vi "Untitled 5.vi"() -> ()   [LabVIEW 2019]
uses:
  <vilib>/Platform/TimedLoop/XDataNode/wakeup.ctl
  <vilib>/Platform/TimedLoop/XDataNode/XDNodeRunTimeDep.lvlib
  <vilib>/Platform/TimedLoop/XDataNode/nitl_modes.ctl
  <vilib>/Platform/TimedLoop/XDataNode/timing_clust.ctl
  <vilib>/Platform/TimedLoop/XDataNode/XDataNode.xnode
  <vilib>/rvi/DataTransferAndStorage/Container/XNode/niFpgaContainer.xnode
  Templates/FPGA Wizard Templates.lvlib
  <vilib>/rvi/interface/RandomDataEmulation/nirviRandomDataFpgaReadWriteTemplate.vi
  <vilib>/NI/Engine Simulation Toolkit (EST)/APU/Shared Settings.ctl
  <vilib>/NI/Engine Simulation Toolkit (EST)/Version Token.ctl
  <vilib>/NI/Engine Simulation Toolkit (EST)/APU/Settings.ctl
  <vilib>/NI/Engine Simulation Toolkit (EST)/APU/Input.ctl
  <vilib>/NI/Engine Simulation Toolkit (EST)/APU/Output.ctl
  <vilib>/NI/Engine Simulation Toolkit (EST)/Analog Replay/Load Input.ctl
  <vilib>/NI/Engine Simulation Toolkit (EST)/Digital Pattern Generation/Load Input.ctl
  <vilib>/NI/Engine Simulation Toolkit (EST)/Directional Speed/Load Input.ctl
panel:
  out "Numeric":fxp<+/-,32,8> format="%#_27g"
  out "Mod1.Monitor":fxp<+/-,24,5>[](array[numeric])
  in  "Crank":T1
  in  "Exhaust CAM":T2
  in  "Intake CAM":T2
  in  "VR Sensor":T3={"Data"=[0, 0, 0, 0, 0, 0, 0, 0, 0, 0, 0, 0, 0, 0, 0, 0], "LoadOffset"=0, "Done"=FALSE}
  in  "Analog Input Loop Timer (uSec)":u32
  out "output.apu 1":T4 caption="output"
  in  "input.apu 1":T5={"desired speed"=0.0, "reset"=TRUE} caption="input"
  in  "settings.apu 1":T6 caption="settings"
  in  "est.version":T7
  in  "shared settings.apu 1":T8 {"start" format="%#.15g"}
  in  "go.apu 1":bool
  in  "Digital Loop Timer (uSec)":u32
  in  "Analog Output Loop Timer (uSec)":u32
  in  "DMA.Enable":bool
  in  "DMA.MinimumSamples":u32 caption="DMA Loop Timer (uSec)"
  out "DMA.Timeout":bool
  in  "DMA.Timeout.Reset":bool
  in  "DMA Loop Timer (uSec)":u32
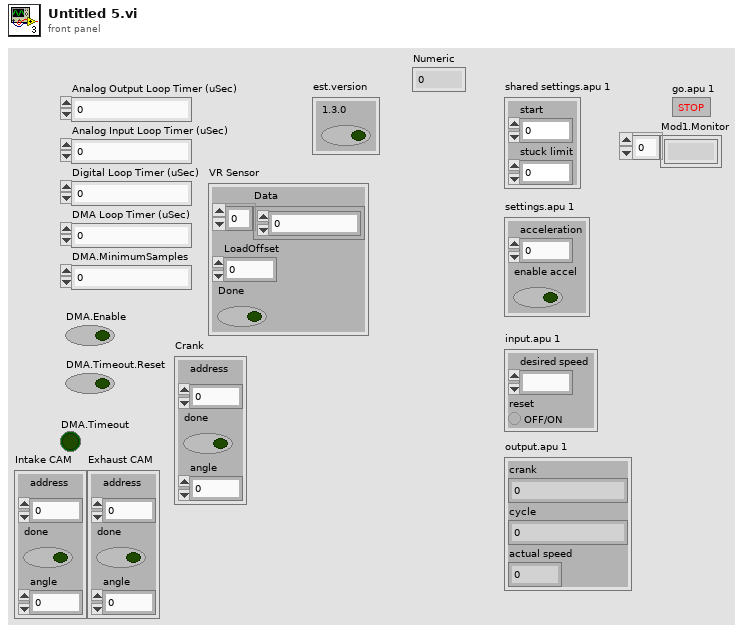
[diagram p1: front panel]
types:
  T1 = typedef "Engine Simulation Toolkit.lvlib/Directional Speed.lvlib/Load Input.ctl" = cluster{"address":fxp<+,10,10>, "done":bool, "angle":u16}
  T2 = typedef "Engine Simulation Toolkit.lvlib/Digital Pattern Generation.lvlib/Load Input.ctl" = cluster{"address":fxp<+,11,11>, "done":bool, "angle":u16}
  T3 = typedef "Engine Simulation Toolkit.lvlib/Analog Replay.lvlib/Load Input.ctl" = cluster{"Data":i16[], "LoadOffset":u16, "Done":bool}
  T4 = typedef "Engine Simulation Toolkit.lvlib/APU.lvlib/Output.ctl" = cluster{"crank":u16, "cycle":u16, "actual speed":fxp<+/-,23,2>}
  T5 = typedef "Engine Simulation Toolkit.lvlib/APU.lvlib/Input.ctl" = cluster{"desired speed":fxp<+/-,23,2>, "reset":bool}
  T6 = typedef "Engine Simulation Toolkit.lvlib/APU.lvlib/Settings.ctl" = cluster{"acceleration":fxp<+,18,-20>, "enable accel":bool}
  T7 = typedef "Engine Simulation Toolkit.lvlib/Version Token.ctl" = cluster{"1.3.0":bool}
  T8 = typedef "Engine Simulation Toolkit.lvlib/APU.lvlib/Shared Settings.ctl" = cluster{"start":fxp<+,17,17>, "stuck limit":fxp<+,18,18>}
  T9 = typedef "XDNodeRunTimeDep.lvlib/timing_clust.ctl" = cluster{"Expected End [f-1]":u64, "Actual End [f-1]":u64, "Finished Late? [f-1]":bool, "Expected End [i-1]":u64, "Actual End [i-1]":u64, "Finished Late? [i-1]":bool, "Expected Start [i]":u64, "Actual Start [i]":u64, "Expected Start [f]":u64, "Actual Start [f]":u64, "Source Name":string, "Structure Name":string, "Period":i64, "Deadline":i64, "Offset":i64, "Start":i64, "Priority":i32, "Timeout":i32, "Mode":T10, "Wakeup Reason":T11, "Error":errorcluster, "Source Type":string, "Secondary Source Type":string, "Global End Time":u64, "Global Start Time":u64, "Frame Duration":u64, "Iteration Duration":u64, "Assigned CPU":i32, "I/O Scan Engine Mode":u32}
  T10 = typedef "XDNodeRunTimeDep.lvlib/nitl_modes.ctl" = enum32{"No Change", "Process missed periods, maintain original phase", "Discard missed periods, maintain original phase", "Process missed periods, ignore original phase", "Discard missed periods, ignore original phase"}
  T11 = typedef "XDNodeRunTimeDep.lvlib/wakeup.ctl" = enum32{"Normal", "Aborted", "Asynchronous wakeup", "Timing source error", "Timed loop error", "Timeout"}
  T12 = cluster{"AI 0":refnum<k21>, "AI 1":refnum<k21>, "AI 2":refnum<k21>, "AI 3":refnum<k21>, "AI 4":refnum<k21>, "AI 5":refnum<k21>, "AI 6":refnum<k21>, "AI 7":refnum<k21>, "AI 8":refnum<k21>, "AI 9":refnum<k21>, "AI 10":refnum<k21>, "AI 11":refnum<k21>, "AI 12":refnum<k21>, "AI 13":refnum<k21>, "AI 14":refnum<k21>, "AI 15":refnum<k21>}
  T13 = typedef "Engine Simulation Toolkit.lvlib/APU.lvlib/Register Bus.ctl" = cluster{"Speed":refnum<k21>, "Crank Angle":refnum<k21>, "Cycle Angle":refnum<k21>, "Crank Count":refnum<k21>, "Cycle Count":refnum<k21>, "1.25 MHz Counter":refnum<k21>, "Crank Rollover":refnum<k21>, "Cycle Rollover":refnum<k21>, "shared settings":T8}
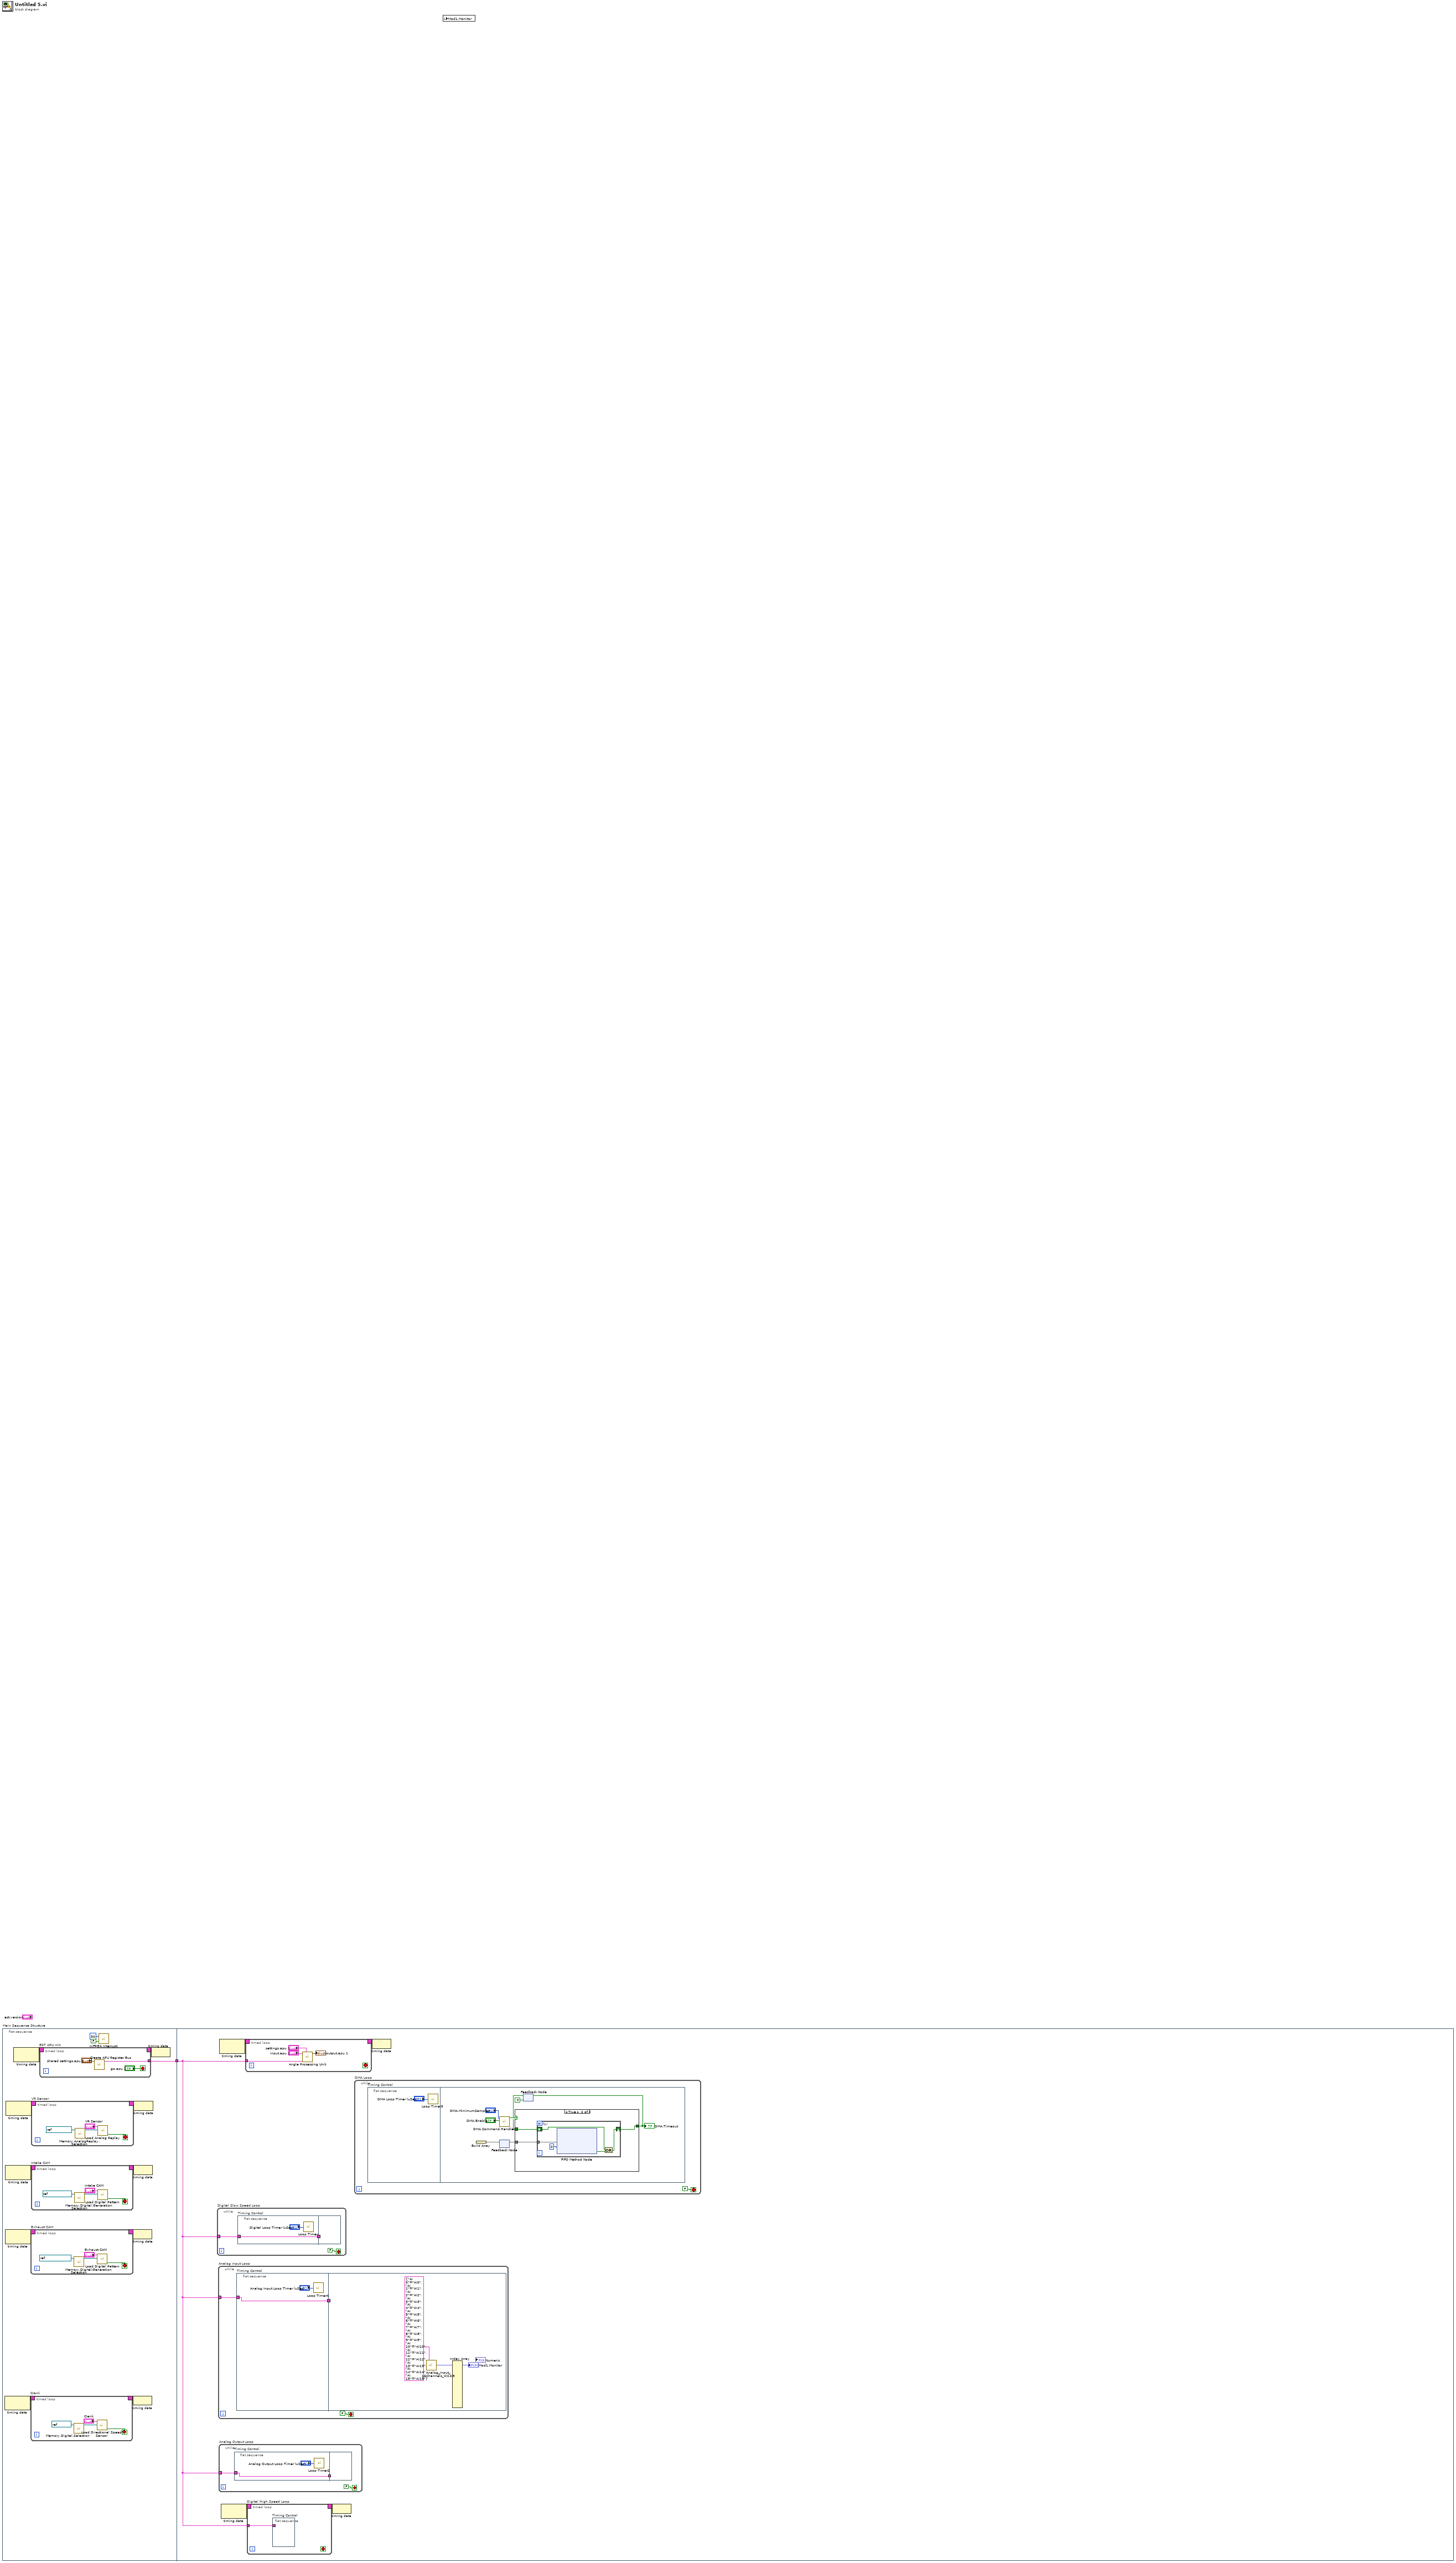
[diagram p0: block diagram]
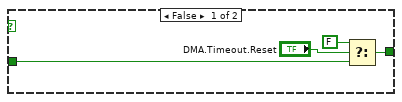
[diagram p2: hidden frame]
diagram:
  n1 = flat-sequence "Main Sequence Structure" {
    tunnel: [w10] -> w1
    tunnel: w1 -> [w54]
    frame #0 {
      n2 = node-c288() -> (w3:T9)  [unwired: 1 in]
      n3 = node-c288() -> (w5:T9)  [unwired: 1 in]
      n4 = node-c288() -> (w7:T9)  [unwired: 1 in]
      n5 = node-c288() -> (w9:T9)  [unwired: 1 in]
      n6 = node-c288() -> (w12:T9)  [unwired: 1 in]
      n7 = timed-loop "Crank" {
        timing: w3 -> [_]
        timing-out: [_] -> w2
        stop <- w17 stop-if-true
        n8 = call "Memory.Digital.Selection.vi"("memory"=refnum<k21> "Crank") -> ("memory"=w15:refnum<k21>)  [unwired: 10 in]
        n9 = call <vilib>:"Load Directional Speed Sensor.vi"("Memory In"=w15, "load input.<user name>"="Crank") -> ("done"=w17:bool)  [unwired: 8 in, 1 out]
      }
      n10 = timed-loop "Exhaust CAM" {
        timing: w5 -> [_]
        timing-out: [_] -> w4
        stop <- w25 stop-if-true
        n11 = call "Memory.Digital.Selection.vi"("memory"=refnum<k21> "Exhaust CAM") -> ("memory"=w23:refnum<k21>)  [unwired: 10 in]
        n12 = call <vilib>:"Load Digital Pattern Generation.vi"("memory"=w23, "load input.<user name>"="Exhaust CAM") -> ("done"=w25:bool)  [unwired: 8 in, 1 out]
      }
      n13 = timed-loop "Intake CAM" {
        timing: w7 -> [_]
        timing-out: [_] -> w6
        stop <- w33 stop-if-true
        n14 = call "Memory.Digital.Selection.vi"("memory"=refnum<k21> "Intake CAM") -> ("memory"=w31:refnum<k21>)  [unwired: 10 in]
        n15 = call <vilib>:"Load Digital Pattern Generation.vi"("memory"=w31, "load input.<user name>"="Intake CAM") -> ("done"=w33:bool)  [unwired: 8 in, 1 out]
      }
      n16 = timed-loop "VR Sensor" {
        timing: w9 -> [_]
        timing-out: [_] -> w8
        stop <- w41 stop-if-true
        n17 = call "Memory.AnalogReplay.Selection.vi"("memory"=refnum<k21> "VR Sensor") -> ("memory"=w39:refnum<k21>)  [unwired: 10 in]
        n18 = call <vilib>:"Load Analog Replay.vi"("memory"=w39, "load input.<user name>"="VR Sensor") -> ("done"=w41:bool)  [unwired: 9 in]
      }
      n19 = timed-loop "EST APU Init" {
        timing: w12 -> [_]
        timing-out: [_] -> w11
        tunnel: [w47] -> w10
        stop <- "go.apu 1" stop-if-true
        n20 = call <vilib>:"Create APU Register Bus.vi"("shared settings.<user name>"="shared settings.apu 1") -> ("register bus"=w47:T13)  [unwired: 10 in]
      }
      n21 = call <vilib>:"niFPGA Interrupt.vi"("Wait Until Cleared (F)"=FALSE, "IRQ Number (0)"=u8 30) -> ()  [unwired: 1 in]
      n22 = node-c288(w2) -> ()
      n23 = node-c288(w4) -> ()
      n24 = node-c288(w6) -> ()
      n25 = node-c288(w8) -> ()
      n26 = node-c288(w11) -> ()
    }
    frame #1 {
      # "FPGA Addon Code"
      n27 = while "Digital Slow Speed Loop" {
        tunnel: w54 -> [w107]
        stop <- FALSE stop-if-true
        n28 = flat-sequence "Timing Control" {
          tunnel: w107 -> [w109]
          tunnel: [w109] -> w106
          tunnel: w106 -> [_]
          frame #0 {
            n29 = call "Loop Timer"("Count(uSec)"="Digital Loop Timer (uSec)") -> ()  [unwired: 1 out]
          }
          frame #1 {
          }
        }
      }
      n30 = while "Analog Input Loop" {
        tunnel: w54 -> [w100]
        stop <- FALSE stop-if-true
        n31 = flat-sequence "Timing Control" {
          tunnel: w100 -> [w102]
          tunnel: [w102] -> w99
          tunnel: w99 -> [_]
          frame #0 {
            n32 = call "Loop Timer4"("Count(uSec)"="Analog Input Loop Timer (uSec)") -> ()  [unwired: 1 out]
          }
          frame #1 {
            n33 = call "Analog_Input_16Channels_W24I5.vi"("IO"=T12 {"AI 0"="AI0", "AI 1"="AI1", "AI 2"="AI2", "AI 3"="AI3", "AI 4"="AI4", "AI 5"="AI5", "AI 6"="AI6", "AI 7"="AI7", "AI 8"="AI8", "AI 9"="AI9", "AI 10"="AI10", "AI 11"="AI11", "AI 12"="AI12", "AI 13"="AI13", "AI 14"="AI14", "AI 15"="AI15"}) -> ("Values"=w104:fxp<+/-,24,5>[])
            "Mod1.Monitor" <- w104
            n34 = Index Array(array=w104) -> ()  [unwired: 16 in, 16 out]
          }
        }
      }
      n35 = while "Analog Output Loop" {
        tunnel: w54 -> [w95]
        stop <- FALSE stop-if-true
        n36 = flat-sequence "Timing Control" {
          tunnel: w95 -> [w97]
          tunnel: [w97] -> w94
          tunnel: w94 -> [_]
          frame #0 {
            n37 = call "Loop Timer2"("Count(uSec)"="Analog Output Loop Timer (uSec)") -> ()  [unwired: 1 out]
          }
          frame #1 {
          }
        }
      }
      n38 = node-c288 ("Input Node")() -> (w56:T9)  [unwired: 1 in]
      n39 = node-c288() -> (w58:T9)  [unwired: 1 in]
      n40 = timed-loop "Timed Loop" {
        timing: w56 -> [_]
        timing-out: [_] -> w55
        tunnel: w54 -> [w59]
        stop <- _ stop-if-true
        n41 = call <vilib>:"Angle Processing Unit.vi"("settings.<user name>"="settings.apu 1", "register bus"=w59, "input.<user name>"="input.apu 1") -> ("output.<user name>"=→"output.apu 1":T4)  [unwired: 8 in]
      }
      n42 = timed-loop "Digital High Speed Loop" {
        timing: w58 -> [_]
        timing-out: [_] -> w57
        tunnel: w54 -> [w67]
        stop <- _ stop-if-true
        n43 = flat-sequence "Timing Control" {
          tunnel: w67 -> [_]
          frame #0 {
          }
        }
      }
      n44 = node-c288 ("Output Node")(w57) -> ()
      n45 = while "DMA Loop" {
        stop <- FALSE stop-if-true
        n46 = flat-sequence "Timing Control" {
          frame #0 {
            n47 = call "Loop Timer3"("Count(uSec)"="DMA Loop Timer (uSec)") -> ()  [unwired: 1 out]
          }
          frame #1 {
            n48 = Build Array "Build Array"() -> (w79:void[])  [unwired: 1 in]
            n49 = call "DMA.Command.Handler.vi"("DMA.Enable"="DMA.Enable", "DMA.MinimumSamples"="DMA.MinimumSamples") -> ("Transfer"=w75:bool)  [unwired: 9 in]
            n50 = feedback #1() -> (w78:void[])  [unwired: 1 in]
            n51 = feedback-in #1(w79) -> ()
            n52 = feedback #2(FALSE ("t")) -> (w74:bool)
            n53 = case shown="True" w75 {
              tunnel: w78 -> [_ w88]
              tunnel: w74 -> [w83 w87]
              tunnel: [w82 w86] -> w77
              frame False {
                n54 = Select(t=FALSE, s="DMA.Timeout.Reset", f=w83) -> (s? t:f=w82:bool)
              }
              frame True {
                n55 = for {
                  shift-right: [w91] -> w86
                  shift-left: w87 -> [w90]
                  tunnel: w88 -> [w89] mode=indexing
                  n56 = xnode ("FIFO Method Node")("Element"=w89, "Timeout"=0) -> ("Timed Out?"=w92:bool)  [unwired: 1 in, 1 out]
                  n57 = Or(x=w90, y=w92) -> (x .or. y?=w91:bool)
                }
              }
            }
            "DMA.Timeout" <- w77
            n58 = feedback-in #2(w77) -> ()
          }
        }
      }
      n59 = node-c288 ("Output Node")(w55) -> ()
    }
  }
  n60 = local read "Mod1.Monitor"() -> ()  [unwired: 1 in]
